vi "writeToXML.vi"(8 "error in (no error)":errorcluster, 10 "ClassLabel":string, 11 "POrigin in":refnum<class "POrigin.lvclass">) -> (0 "error out":errorcluster, 2 "XML out":string, 3 "POrigin out":refnum<class "POrigin.lvclass">)   [LabVIEW 2014, in "TCSDataDefinitions.lvlib" / "TCSCommand.lvlib" / "POriginCommands.lvlib" / "POrigin.lvclass"]
uses:
  POrigin.lvclass
  <userlib>/Common/UnitsAndXML/FlattenItemWithUnitToXML/FlattenLengthToXML/LengthUnit.ctl
  POrigin.lvclass/POrigin.ctl
  POriginCommands/POriginCommands.lvclass
  <userlib>/Common/UnitsAndXML/UnitsAndXML.lvlib
  <userlib>/Common/XML/XMLGenerator/XMLGenerator.lvclass
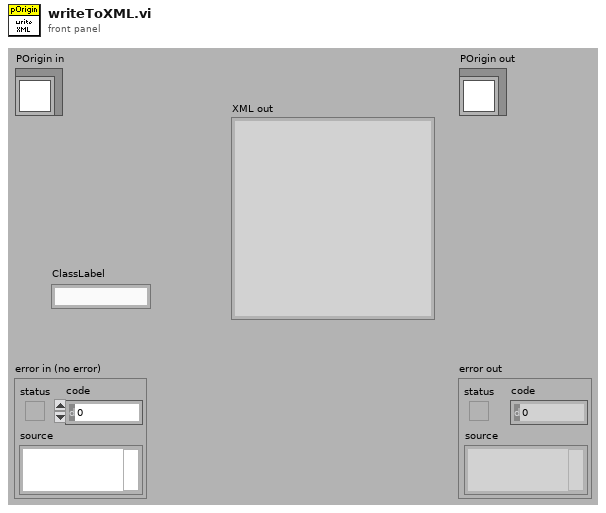
[diagram p1: front panel]
types:
  T1 = typedef "UnitsAndXML.lvlib/LengthUnit.ctl" = enum16{"m", "Angstrom", "AU", "chain", "cm", "cubit", "fathom", "fermi", "ft", "furlong", "hubble", "in", "ly", "mi", "mm", "rod", "um", "yd"}
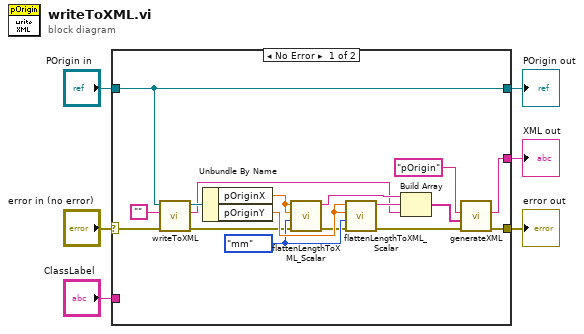
[diagram p0: block diagram]
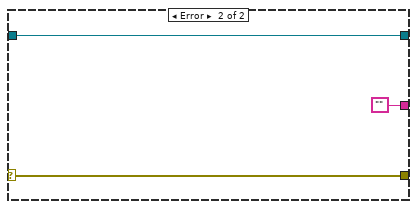
[diagram p2: hidden frame]
diagram:
  n1 = case shown="No Error" "error in (no error)" {
    selector: "error in (no error)" -> [w21 w26]
    tunnel: [w9 w26] -> w5
    tunnel: [w23 w25] -> w3
    tunnel: "POrigin in" -> [w23 w25]
    tunnel: [w8 ""] -> w2
    tunnel: "ClassLabel" -> [_ _]
    frame No Error {
      w18 = LengthUnit."mm" ("lengthUnitInXML")
      n2 = call-parent "writeToXML.vi"("error in (no error)"=w21, "ClassLabel"="", "POriginCommands in"=w23) -> ("error out"=w10:errorcluster, "XML out"=w14:string, "POriginCommands out"=w22:refnum<class "POrigin.lvclass">)  [unwired: 6 in]
      n3 = Unbundle By Name(w22) -> ("pOriginX"=w20:dbl[unit], "pOriginY"=w19:dbl[unit])
      n4 = call <userlib>:"flattenLengthToXML_Scalar.vi"("error in (no error)"=w10, "lengthUnitInXML"=w18, "lengthAgain"=w20, "length"=w20) -> ("error out"=w17:errorcluster, "xmlString"=w16:string)  [unwired: 6 in]
      n5 = call <userlib>:"flattenLengthToXML_Scalar.vi"("error in (no error)"=w17, "lengthUnitInXML"=w18, "lengthAgain"=w19, "length"=w19) -> ("error out"=w11:errorcluster, "xmlString"=w15:string)  [unwired: 6 in]
      n6 = Build Array(w16, w15, w14) -> (w13:string[])
      n7 = call <userlib>:"generateXML.vi"("error in"=w11, "childrenXML"=w13, "elementName"="pOrigin" ("Class Label")) -> ("error out"=w9:errorcluster, "XML out"=w8:string)  [unwired: 6 in, 1 out]
    }
    frame Error {
    }
  }
  "error out" <- w5
  "POrigin out" <- w3
  "XML out" <- w2
